vi "sensorNameToFieldIdx.vi"(8 "error in (no error)":errorcluster, 9 "Sensor Name":string, 10 "Path":path=path "/home/ttsai/Documents/stash/ts_tcs_ofc/configData/lsst/sensorNameToFieldIdx.txt", 11 "MatOper in":refnum<class "MatOper.lvclass">) -> (0 "error out":errorcluster, 2 "Idx of Field":i32, 3 "MatOper out":refnum<class "MatOper.lvclass">)   [LabVIEW 2016, in "OfcFunc.lvlib" / "MatOper.lvclass"]
doc: "Transfer the abbreviate sensor name (e.g. R22_S11) to the index of optical field."
uses:
  MatOper.lvclass
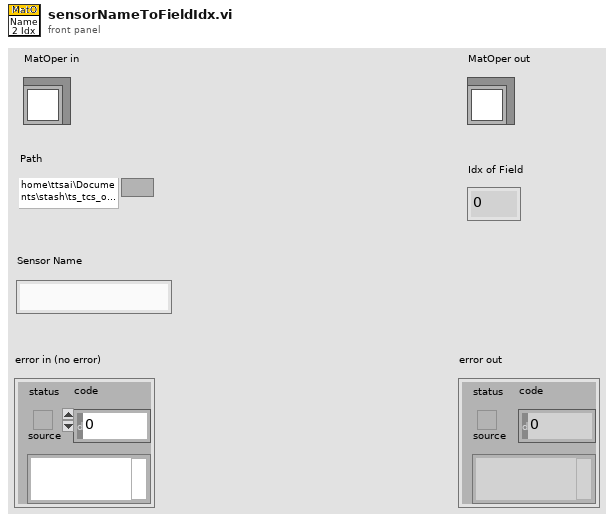
[diagram p1: front panel]
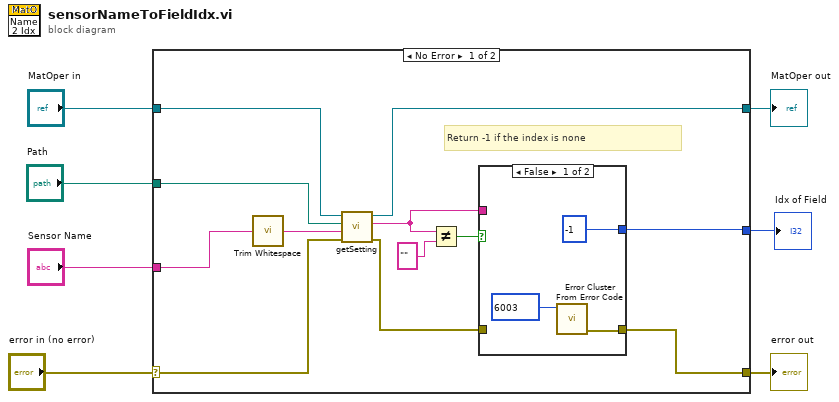
[diagram p0: block diagram]
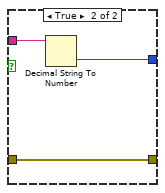
[diagram p2: hidden frame]
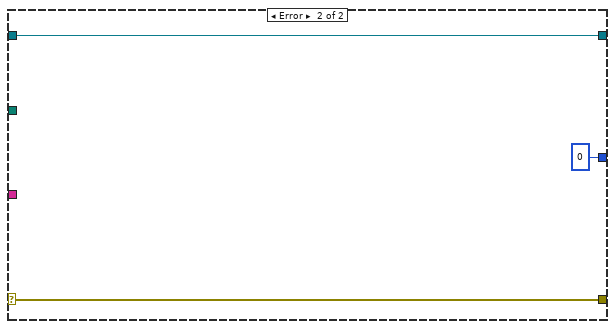
[diagram p3: hidden frame]
diagram:
  n1 = case shown="No Error" "error in (no error)" {
    selector: "error in (no error)" -> [w13 w28]
    tunnel: [w14 w28] -> w6
    tunnel: [w8 w27] -> w4
    tunnel: "MatOper in" -> [w9 w27]
    tunnel: [w12 0] -> w3
    tunnel: "Sensor Name" -> [w11 _]
    tunnel: "Path" -> [w10 _]
    frame No Error {
      # "Return -1 if the index is none"
      n2 = call <vilib>:"Trim Whitespace.vi"("string"=w11) -> ("trimmed string"=w19:string)  [unwired: 1 in]
      n3 = call "getSetting.vi"("error in (no error)"=w13, "Parameter"=w19, "Path"=w10, "MatOper in"=w9) -> ("error out"=w15:errorcluster, "Value"=w17:string, "MatOper out"=w8:refnum<class "MatOper.lvclass">)  [unwired: 5 in]
      n4 = Not Equal?(x=w17, y="") -> (x != y?=w16:bool)
      n5 = case shown="False" w16 {
        tunnel: w17 -> [_ w25]
        tunnel: [-1 w24] -> w12
        tunnel: w15 -> [_ w23]
        tunnel: [w20 w23] -> w14
        frame False {
          n6 = call <vilib>:"Error Cluster From Error Code.vi"("error code (0)"=6003 ("code")) -> ("error out"=w20:errorcluster)  [unwired: 8 in]
        }
        frame True {
          n7 = Decimal String To Number(string=w25) -> (number=w24:i32)  [unwired: 2 in, 1 out]
        }
      }
    }
    frame Error {
    }
  }
  "error out" <- w6
  "MatOper out" <- w4
  "Idx of Field" <- w3
